vi "Phase Feedback Cluster.vi"() -> ()   [LabVIEW 2018]
uses:
  Phase Calculator Feedback Cluster.ctl
panel:
  in  "Cluster":T1
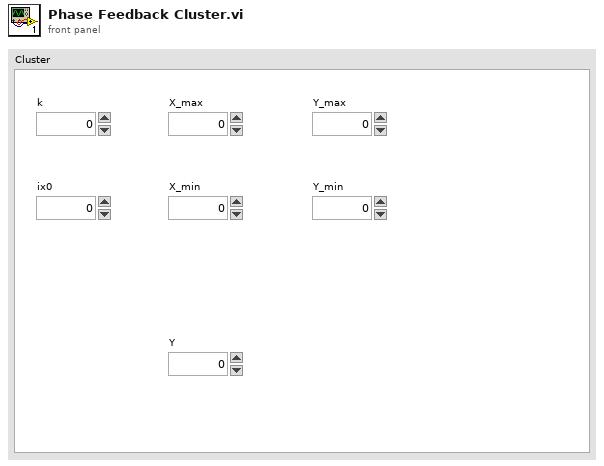
[diagram p1: front panel]
types:
  T1 = typedef "Phase Calculator Feedback Cluster.ctl" = cluster{"k":dbl, "ix0":dbl, "X_max":dbl, "X_min":dbl, "Y_max":dbl, "Y_min":dbl, "Y":dbl}
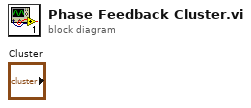
[diagram p0: block diagram]
diagram:
